vi "Allow Undefined.vi"(8 "error in (no error)":errorcluster, 11 "Shared Options in":refnum<class "Shared Options.lvclass">) -> (0 "error out":errorcluster, 2 "Allow Undefined Values":bool, 3 "Shared Options out":refnum<class "Shared Options.lvclass">)   [LabVIEW 2020, in "AutoComplete.lvlib" / "Shared Options.lvclass"]
uses:
  Shared Options.lvclass
  Shared Options.lvclass/Shared Options.ctl
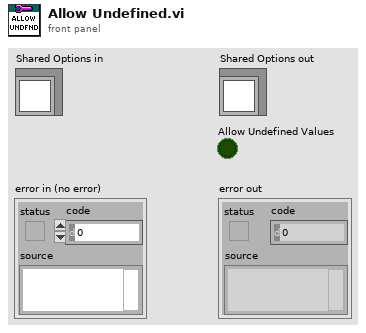
[diagram p1: front panel]
types:
  T1 = typedef "AutoComplete.lvlib/Options.ctl" = cluster{"Options":string[], "Allow Undefined Values":bool}
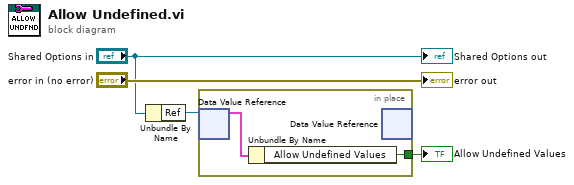
[diagram p0: block diagram]
diagram:
  n1 = Unbundle By Name("Shared Options in") -> ("Ref"=w3:refnum<data-value>)
  n2 = in-place {
    in-place-border: [w5] -> w1
    n3 = in-place-dvr #1(w3) -> (w6:T1)  [unwired: 1 out]
    n4 = Unbundle By Name(w6) -> ("Allow Undefined Values"=w5:bool)
    n5 = in-place-dvr #1() -> ()  [unwired: 1 in, 2 out]
  }
  "Allow Undefined Values" <- w1
  "error out" <- "error in (no error)"
  "Shared Options out" <- "Shared Options in"
